vi "_Remote Update DC.vi"(5 "DC Inputs":string[][](array[string]), 6 "Table Reference":refnum<vi>, 7 "Ch#":u8[](array[numeric])=[4, 7, 6]) -> (1 "DC Outputs":string[][](array[string]), 2 "Total":dbl, 3 "VDC":dbl)   [LabVIEW 2012]
uses:
  Type/_RT Active Ch.ctl
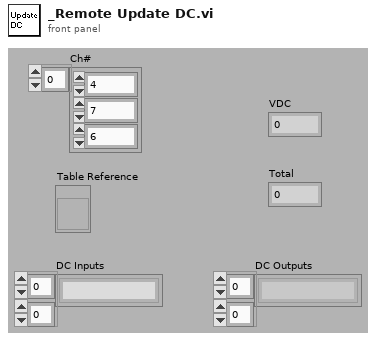
[diagram p1: front panel]
types:
  T1 = typedef "_RT Active Ch.ctl" = cluster{"Start":i32, "Step":i32, "ChID":i32}
  T2 = typedef "_RT Configuration 2.ctl" = cluster{"Name":string, "Ch#":u8, "Min":dbl, "Max":dbl, "Def+":dbl, "Def-":dbl, "Offset":dbl, "Slope":dbl, "Type":u8, "Description":string, "SettleT":dbl}
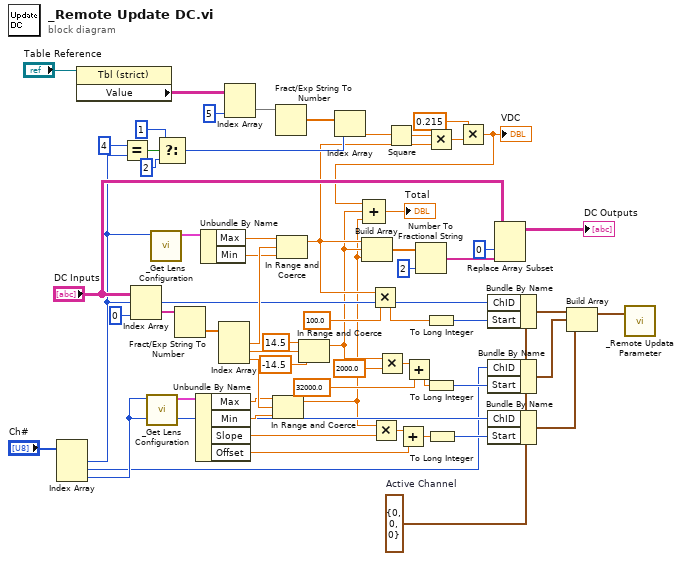
[diagram p0: block diagram]
diagram:
  w61 = T1 {"Start"=0, "Step"=0, "ChID"=0}  # Active Channel
  n1 = Index Array(array="Ch#") -> (element #1=w15:u8, element #2=w25:u8, element #3=w26:u8)  [unwired: 3 in]
  n2 = property class="Tbl (strict)"(reference="Table Reference") -> ("Value"=w18:string[][])  [unwired: 1 in, 2 out]
  n3 = Equal?(x=u8 4, y=w15) -> (x = y?=w13:bool)
  n4 = Index Array(array="DC Inputs", index (col)=0 ("disabled index (col)")) -> (element=w29:string[])  [unwired: 1 in]
  n5 = call "_Get Lens Configuration.vi"("Channel #"=w26) -> ("Lens Configuration"=w40:T2)  [unwired: 1 in, 5 out]
  n6 = call "_Get Lens Configuration.vi"("Channel #"=w15) -> ("Lens Configuration"=w34:T2)  [unwired: 1 in, 5 out]
  n7 = Select(t=1 ("dimension size"), s=w13, f=2) -> (s? t:f=w10:i32)
  n8 = Fract/Exp String To Number(string=w29) -> (number=w30:dbl[])  [unwired: 4 out]
  n9 = Unbundle By Name(w40) -> ("Max"=w39:dbl, "Min"=w38:dbl, "Slope"=w52:dbl, "Offset"=w53:dbl)
  n10 = Unbundle By Name(w34) -> ("Max"=w35:dbl, "Min"=w36:dbl)
  n11 = Index Array(array=w30) -> (element #1=w37:dbl, element #2=w31:dbl, element #3=w41:dbl)  [unwired: 3 in]
  n12 = Index Array(array=w18, index (col)=5 ("disabled index (col)")) -> (element=w16:string[])  [unwired: 1 in]
  n13 = In Range and Coerce(upper limit=w39, x=w41, lower limit=w38) -> (coerced(x)=w2:dbl)  [unwired: 1 out]
  n14 = Fract/Exp String To Number(string=w16) -> (number=w17:dbl[])  [unwired: 4 out]
  n15 = In Range and Coerce(upper limit=w35, x=w37, lower limit=w36) -> (coerced(x)=w5:dbl)  [unwired: 1 out]
  n16 = In Range and Coerce(upper limit=14.5, x=w31, lower limit=-14.5) -> (coerced(x)=w3:dbl)  [unwired: 1 out]
  n17 = Index Array(array=w17, index=w10) -> (element=w9:dbl)
  n18 = Build Array(w5, w3, w2) -> (w42:dbl[])
  n19 = Multiply(x=w5, y=100.0) -> (x*y=w49:dbl)
  n20 = Multiply(x=w2, y=w52) -> (x*y=w51:dbl)
  n21 = Multiply(x=w3, y=2000.0) -> (x*y=w57:dbl)
  n22 = Square(x=w9) -> (x^2=w8:dbl)
  n23 = Add(x=w51, y=w53) -> (x+y=w55:dbl)
  n24 = Add(x=w57, y=32000.0) -> (x+y=w60:dbl)
  n25 = Number To Fractional String(number=w42, precision (6)=i16 2) -> (F-format string=w46:string[])  [unwired: 2 out]
  n26 = Multiply(x=w8, y=w5) -> (x*y=w7:dbl)
  n27 = To Long Integer(number=w49) -> (32bit integer=w50:i32)
  n28 = To Long Integer(number=w60) -> (32bit integer=w56:i32)
  n29 = To Long Integer(number=w55) -> (32bit integer=w54:i32)
  n30 = Multiply(x=0.215, y=w7) -> (x*y=w4:dbl)
  "VDC" <- w4
  n31 = Compound Arithmetic op=ADD(w4, w3, w2) -> (→"Total":dbl)
  n32 = Bundle By Name(cluster=w61, "ChID"=w15, "Start"=w50) -> (w24:T1)
  n33 = Bundle By Name(cluster=w61, "ChID"=w25, "Start"=w56) -> (w23:T1)
  n34 = Bundle By Name(cluster=w61, "ChID"=w26, "Start"=w54) -> (w22:T1)
  n35 = Replace Array Subset(array="DC Inputs", new element=w46, index (col)=0 ("disabled index (col)")) -> (→"DC Outputs":string[][])  [unwired: 1 in]
  n36 = Build Array(w24, w23, w22) -> (w21:T1[])
  n37 = call "_Remote Updata Parameter.vi"("Parameters"=w21) -> ()  [unwired: 1 in, 1 out]
